vi "Verify that types are supported.vi"(8 "error in":errorcluster, 11 "Section (Cluster)":variant) -> (0 "error out":errorcluster, 3 "Section (Cluster)":variant)   [LabVIEW 2024, in "Generic Config Handling.lvlib"]
doc: "This vi is used to check that the cluster variant passed is in meets the type requirements for this particular library.\n\nThis library only supports certain datatypes. If the data is not of the correct type it will generate an error 999."
uses:
  Generic Config Handling.lvlib
  <vilib>/Utility/VariantDataType/VariantType.lvlib
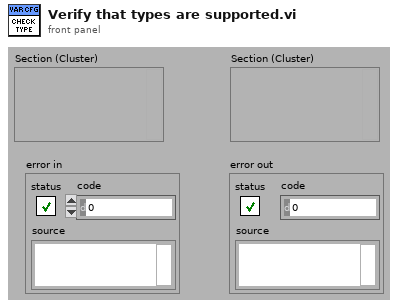
[diagram p1: front panel]
types:
  T1 = typedef "VariantType.lvlib/Type.ctl" = enum8{"Invalid Type", "Void", "I8", "I16", "I32", "I64", "U8", "U16", "U32", "U64", "Single Float", "Double Float", "Extended Float", "Single Complex", "Double Complex", "Extended Complex", "Enum U8", "Enum U16", "Enum U32", "Enum U64", "Single Float With Unit", "Double Float With Unit", "Extended Float With Unit", "Single Complex with Unit", "Double Complex with Unit", "Extended Complex with Unit", "Boolean", "String", "Path", "Picture", "Tag", "Array", "Cluster", "Variant", "LV Variant", "Waveform", "Timestamp", "Digital Waveform", "Digital Data", "ExpressData", "Refnum", "External Data", "VI", "Poly VI", "LabVIEW Class Instance", "Fixed Point"}
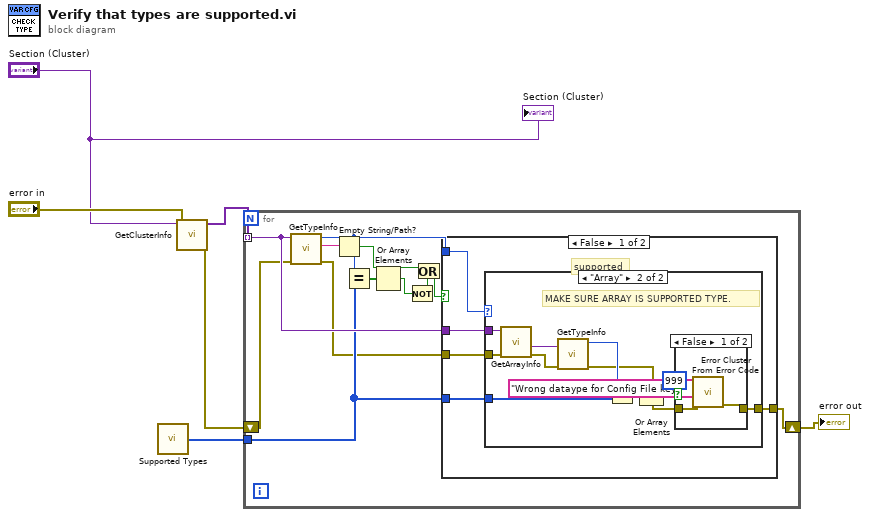
[diagram p0: block diagram]
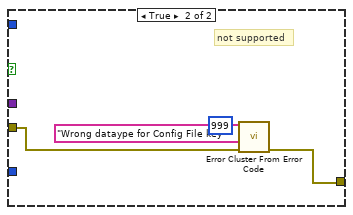
[diagram p4: hidden frame]
diagram:
  n1 = call "Supported Types.vi"() -> ("Supported Types"=w4:T1[])
  n2 = call <vilib>:"GetClusterInfo.vi"("error in (no error)"="error in", "Variant"="Section (Cluster)") -> ("error out"=w3:errorcluster, "Cluster Elements"=w6:variant[])  [unwired: 8 in]
  n3 = for {
    tunnel: w6 -> [w15] mode=indexing
    shift-right: [w11] -> w5
    shift-left: w3 -> [w13]
    tunnel: w4 -> [w14]
    n4 = call <vilib>:"GetTypeInfo.vi"("error in (no error)"=w13, "Variant"=w15) -> ("error out"=w12:errorcluster, "Name"=w10:string, "Type Enum"=w16:T1)  [unwired: 5 in, 2 out]
    n5 = Empty String/Path?(string/path=w10) -> (empty?=w8:bool)
    n6 = Equal?(x=w16, y=w14) -> (x = y?=w18:bool[])
    n7 = Or Array Elements(Boolean array=w18) -> (logical OR=w17:bool)
    n8 = Not(x=w17) -> (.not. x?=w9:bool)
    n9 = Or(x=w8, y=w9) -> (x .or. y?=w7:bool)
    n10 = case shown="False" w7 {
      tunnel: w16 -> [w23 _]
      tunnel: w15 -> [w22 _]
      tunnel: w14 -> [w21 _]
      tunnel: w12 -> [w20 w42]
      tunnel: [w19 w41] -> w11
      frame False {
        n11 = case shown="\"Array\"" w23 {
          tunnel: w22 -> [_ w34]
          tunnel: w21 -> [_ w30]
          tunnel: w20 -> [w24 w28]
          tunnel: [w24 w25] -> w19
          frame "Invalid Type", Default {
          }
          frame "Array" {
            # "MAKE SURE ARRAY IS SUPPORTED TYPE."
            # "supported"
            n12 = call <vilib>:"GetArrayInfo.vi"("error in (no error)"=w28, "Variant"=w34) -> ("error out"=w27:errorcluster, "ArrayElement"=w32:variant)  [unwired: 6 in, 2 out]
            n13 = call <vilib>:"GetTypeInfo.vi"("error in (no error)"=w27, "Variant"=w32) -> ("error out"=w26:errorcluster, "Type Enum"=w31:T1)  [unwired: 5 in, 3 out]
            n14 = Equal?(x=w31, y=w30) -> (x = y?=w33:bool[])
            n15 = Or Array Elements(Boolean array=w33) -> (logical OR=w29:bool)
            n16 = case shown="False" w29 {
              tunnel: w26 -> [w37 w39]
              tunnel: [w35 w39] -> w25
              frame False {
                n17 = call <vilib>:"Error Cluster From Error Code.vi"("error in (no error)"=w37, "error message (\"\")"="Wrong dataype for Config File key" ("error message (\"\")"), "error code (0)"=999) -> ("error out"=w35:errorcluster)  [unwired: 6 in]
              }
              frame True {
              }
            }
          }
        }
      }
      frame True {
        # "not supported"
        n18 = call <vilib>:"Error Cluster From Error Code.vi"("error in (no error)"=w42, "error message (\"\")"="Wrong dataype for Config File key" ("error message (\"\")"), "error code (0)"=999) -> ("error out"=w41:errorcluster)  [unwired: 6 in]
      }
    }
  }
  "error out" <- w5
  "Section (Cluster)" <- "Section (Cluster)"
